vi "Get Old Avg.vi"(8 "Error In":errorcluster, 11 "GEA2 Reference In":refnum<k24>) -> (0 "Error Out":errorcluster, 1 "ERD Data Out":T1[](array[typedef]) {"ERD Number" format="%.0x"}, 3 "GEA2 Reference Out":refnum<k24>)   [LabVIEW 2016]
uses:
  Q:/Common/DLLs/GEA3/GeaCommunication.dll
  Common/DLLs/GEA3/GeaCommunication.dll
  Common/LabVIEW GEA2 Toolkit/LabVIEW_GEA2_Toolkit.lvlibp/type defs/ERD Read Data Out.ctl
  Common/LabVIEW GEA2 Toolkit/LabVIEW_GEA2_Toolkit.lvlibp/type defs/Source_Destination.ctl
  Common/LabVIEW GEA2 Toolkit/LabVIEW_GEA2_Toolkit.lvlibp/type defs/ERD Read Data In.ctl
  Common/LabVIEW GEA2 Toolkit/LabVIEW_GEA2_Toolkit.lvlibp/type defs/Data Type.ctl
  Common/LabVIEW GEA2 Toolkit/LabVIEW_GEA2_Toolkit.lvlibp
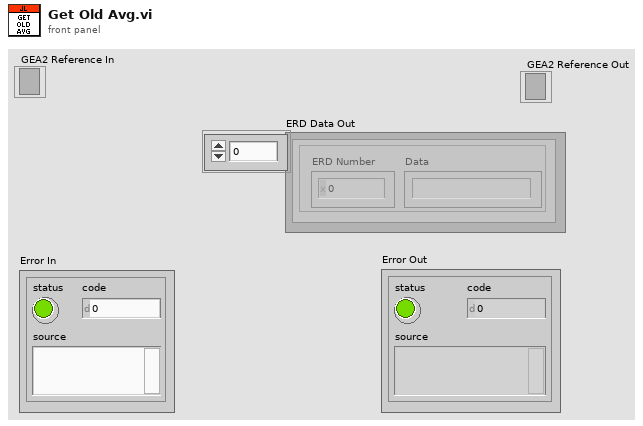
[diagram p1: front panel]
types:
  T1 = typedef "LabVIEW_GEA2_Toolkit.lvlibp/ERD Read Data Out.ctl" = cluster{"ERD Number":u16, "Data":string}
  T2 = typedef "LabVIEW_GEA2_Toolkit.lvlibp/ERD Read Data In.ctl" = cluster{"ERD Number":u16, "Data Type":T3}
  T3 = typedef "LabVIEW_GEA2_Toolkit.lvlibp/Data Type.ctl" = enum16{"string", "boolean", "uint8_t", "uint16_t", "uint32_t", "uint64_t", "int8_t", "int16_t", "int32_t", "int64_t"}
  T4 = typedef "LabVIEW_GEA2_Toolkit.lvlibp/Source_Destination.ctl" = cluster{"Source":u8, "Destination":u8}
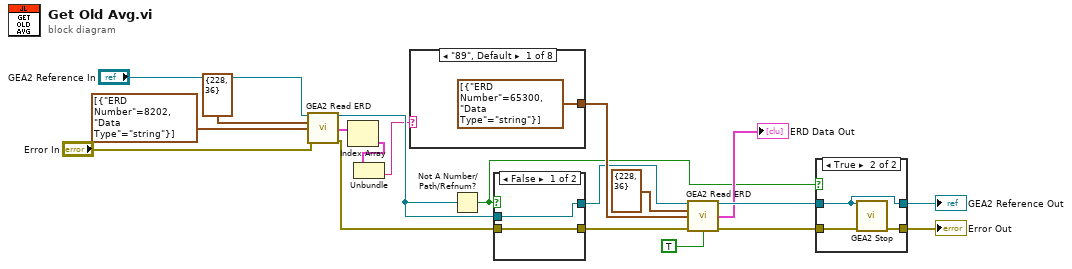
[diagram p0: block diagram]
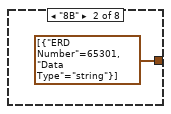
[diagram p2: hidden frame]
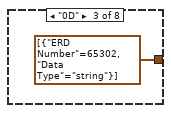
[diagram p3: hidden frame]
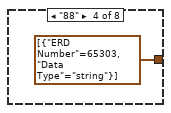
[diagram p4: hidden frame]
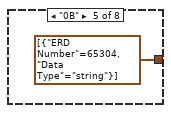
[diagram p5: hidden frame]
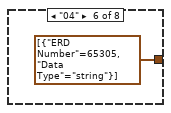
[diagram p6: hidden frame]
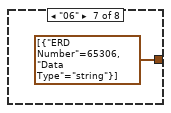
[diagram p7: hidden frame]
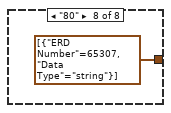
[diagram p8: hidden frame]
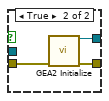
[diagram p10: hidden frame]
diagram:
  n1 = call "GEA2 Read ERD.vi"("GEA2 Reference In"="GEA2 Reference In", "GEA Inputs"=T4 {"Source"=228, "Destination"=36}, "Read ERD List"=T2[] [{"ERD Number"=8202, "Data Type"=enum."string"}], "Error In"="Error In") -> ("GEA2 Reference Out"=w4:refnum<k24>, "ERD Data Out"=w3:T1[], "Error Out"=w6:errorcluster)  [unwired: 8 in, 1 out]
  n2 = Index Array(array=w3) -> (element=w2:T1)  [unwired: 1 in]
  n3 = Unbundle(w2) -> ("Data"=w1:string)  [unwired: 1 out]
  n4 = case shown="\"89\", Default" w1 {
    tunnel: [T2[] [{"ERD Number"=65300, "Data Type"=enum."string"}] ("Read ERD List") T2[] [{"ERD Number"=65301, "Data Type"=enum."string"}] ("Read ERD List") T2[] [{"ERD Number"=65302, "Data Type"=enum."string"}] ("Read ERD List") T2[] [{"ERD Number"=65303, "Data Type"=enum."string"}] ("Read ERD List") T2[] [{"ERD Number"=65304, "Data Type"=enum."string"}] ("Read ERD List") T2[] [{"ERD Number"=65305, "Data Type"=enum."string"}] ("Read ERD List") T2[] [{"ERD Number"=65306, "Data Type"=enum."string"}] ("Read ERD List") T2[] [{"ERD Number"=65307, "Data Type"=enum."string"}] ("Read ERD List")] -> w20
    frame "89", Default {
    }
    frame "8B" {
    }
    frame "0D" {
    }
    frame "88" {
    }
    frame "0B" {
    }
    frame "04" {
    }
    frame "06" {
    }
    frame "80" {
    }
  }
  n5 = Not A Number/Path/Refnum?(number/path/refnum=w4) -> (NaN/Path/Refnum?=w10:bool)
  n6 = case shown="False" w10 {
    tunnel: [w29 w33] -> w12
    tunnel: w6 -> [w29 w32]
    tunnel: [w30 w31] -> w17
    tunnel: w4 -> [w30 _]
    frame False {
    }
    frame True {
      n7 = call "GEA2 Initialize.vi"("error in"=w32) -> ("GEA2 Reference Out"=w31:refnum<k24>, "error out"=w33:errorcluster)  [unwired: 12 in, 1 out]
    }
  }
  n8 = call "GEA2 Read ERD.vi"("GEA2 Reference In"=w17, "GEA Inputs"=T4 {"Source"=228, "Destination"=36}, "Read ERD List"=w20, "Error In"=w12, "Verify ERD Response?"=TRUE) -> ("GEA2 Reference Out"=w16:refnum<k24>, "ERD Data Out"=→"ERD Data Out":T1[], "Error Out"=w18:errorcluster)  [unwired: 7 in, 1 out]
  n9 = case shown="True" w10 {
    tunnel: w18 -> [w34 w38]
    tunnel: [w34 w37] -> w15
    tunnel: [w35 w36] -> w13
    tunnel: w16 -> [w35 w36]
    frame False {
    }
    frame True {
      n10 = call "GEA2 Stop.vi"("GEA2 Reference In"=w36, "Error In"=w38) -> ("Error Out"=w37:errorcluster)  [unwired: 13 in]
    }
  }
  "Error Out" <- w15
  "GEA2 Reference Out" <- w13
